vi "UI_PC event.vi"() -> ()   [LabVIEW 2016]
panel:
  out "RT TCP Loop time 3":u32
  out "RT TCP Loop time 2":u32
  out "RT TCP Loop time":u32
  in  "latch":bool
  in  "type 2":T1
  in  "switch":bool
  in  "정지":bool
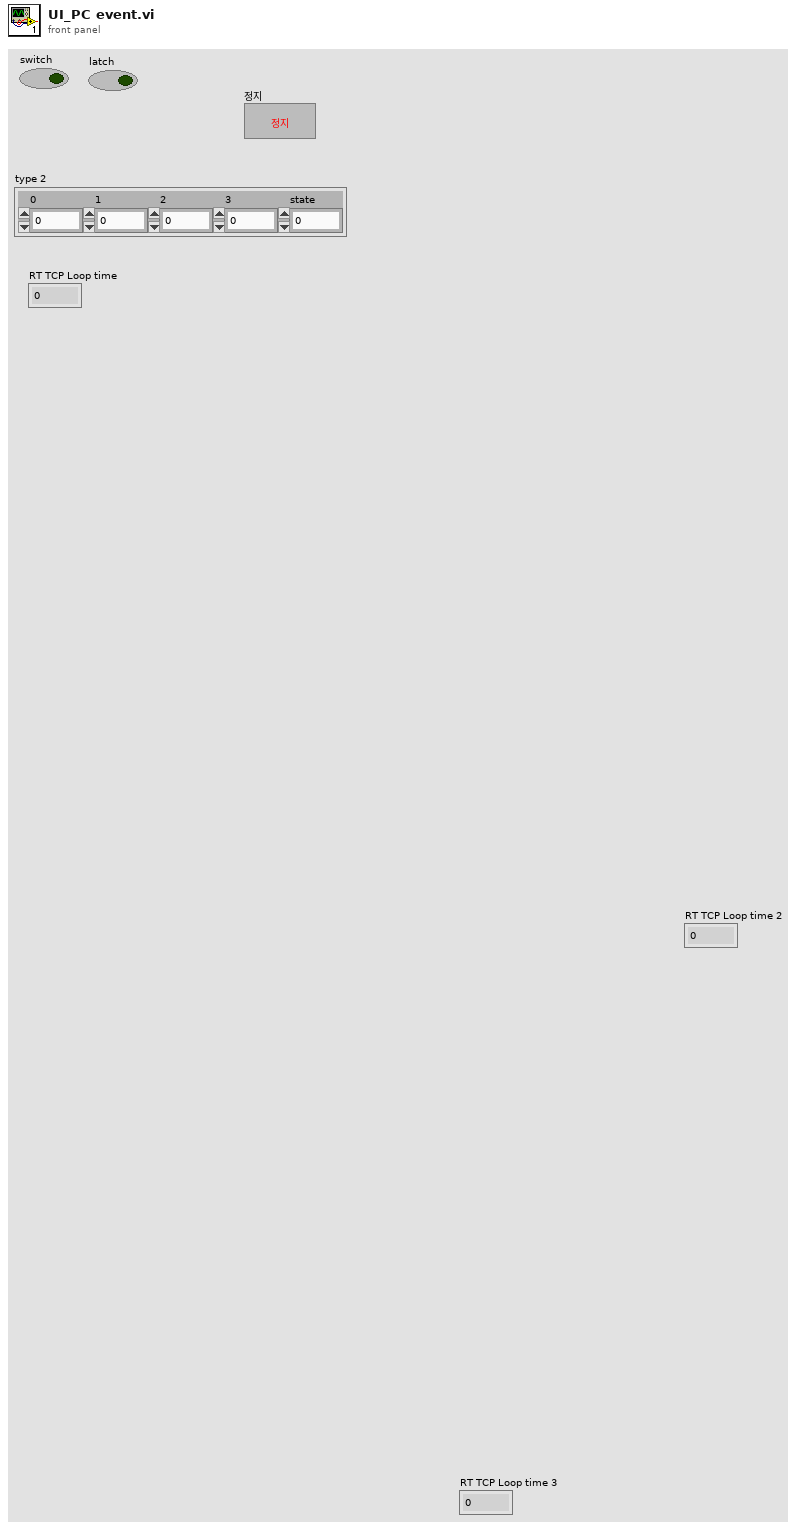
[diagram p1: front panel]
types:
  T1 = cluster{"0":sgl, "1":sgl, "2":sgl, "3":sgl, "state":i32}
  T2 = enum16{"big-endian, network order", "native, host order", "little-endian"}
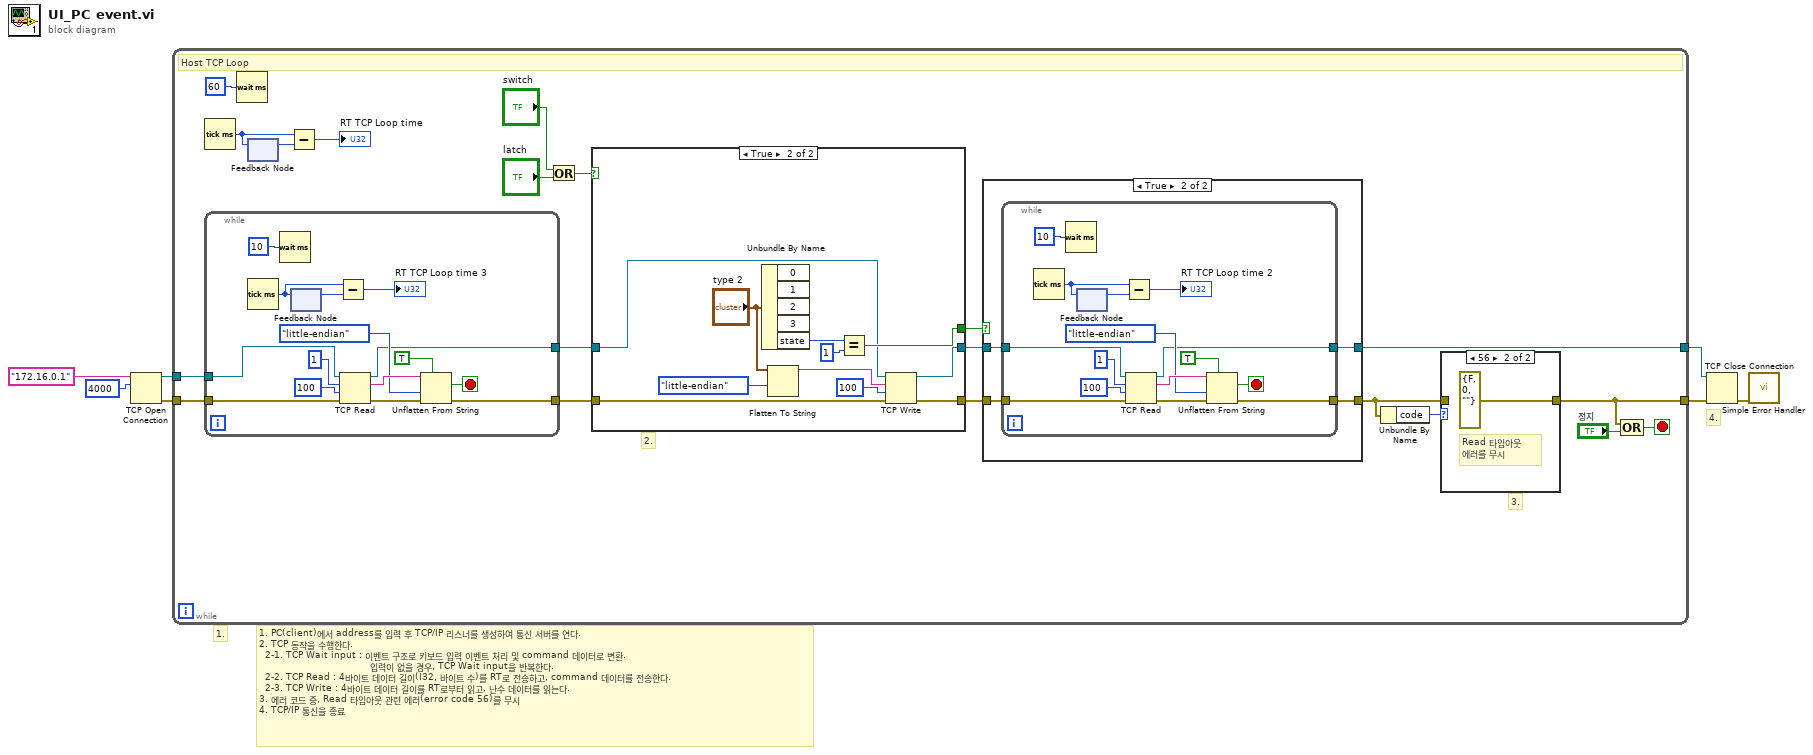
[diagram p0: block diagram]
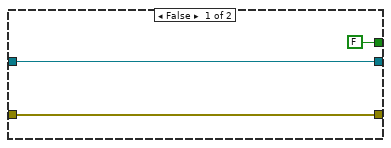
[diagram p3: hidden frame]
diagram:
  # "1. PC(client)에서 address를 입력 후 TCP/IP 리스너를 생성하여 통신 서버를 연다.\n2. TCP 동작을 수행한다.\n  2-1. TCP Wait input : 이벤트 구조로 키보드 입력 이벤트 처리 및 command 데이터로 변환.\n                                     입력이 없을 경우, TCP Wait input을 반복한다.\n  2-2. TCP Read : 4바이트 데이터 길이(I32, 바이트 수)를 RT로 전송하고, command 데이터를 전송한다.\n  2-3. TCP Write : 4바이트 데이터 길이를 RT로부터 읽고, 난수 데이터를 읽는다.\n3. 에러 코드 중, Read 타임아웃 관련 에러(error code 56)를 무시\n4. TCP/IP 통신을 종료"
  # "4."
  # "1."
  n1 = TCP Open Connection(address="172.16.0.1" ("주소"), remote port or service name=u16 4000 ("원격 포트 또는 서비스 이름")) -> (connection ID=w7:refnum<k5>, error out=w4:errorcluster)  [unwired: 3 in]
  n2 = while {
    tunnel: w7 -> [w11]
    tunnel: w4 -> [w10]
    tunnel: [w15] -> w3
    tunnel: [w24] -> w2
    stop <- w26 stop-if-true
    # "2."
    # "3."
    # "Host TCP Loop"
    n3 = Tick Count (ms)() -> (millisecond timer value=w13:u32)
    n4 = while {
      tunnel: w11 -> [w42]
      tunnel: [w34] -> w8
      tunnel: w10 -> [w41]
      tunnel: [w28] -> w9
      stop <- w29 stop-if-true
      n5 = Tick Count (ms)() -> (millisecond timer value=w32:u32)
      n6 = Wait (ms)(milliseconds to wait=u32 10 ("대기 시간 (ms)")) -> ()  [unwired: 1 out]
      n7 = feedback #1() -> (w33:u32)  [unwired: 1 in]
      n8 = feedback-in #1(w32) -> ()
      n9 = Subtract(x=w32, y=w33) -> (x-y=→"RT TCP Loop time 3":u32)
      n10 = TCP Read(connection ID=w42, bytes to read=1, error in (no error)=w41, 9:100 ("타임아웃 ms (25000)")) -> (connection ID out=w34:refnum<k5>, data out=w38:string, error out=w35:errorcluster)  [unwired: 1 in]
      n11 = Unflatten From String(type=TRUE, binary string=w38, byte order (0:big-endian, network order)=T2."little-endian", error in (no error)=w35) -> (value=w29:bool, error out=w28:errorcluster)  [unwired: 1 in, 1 out]
    }
    n12 = Wait (ms)(milliseconds to wait=u32 60 ("대기 시간 (ms)")) -> ()  [unwired: 1 out]
    n13 = feedback #2() -> (w14:u32)  [unwired: 1 in]
    n14 = feedback-in #2(w13) -> ()
    n15 = Subtract(x=w13, y=w14) -> (x-y=→"RT TCP Loop time":u32)
    n16 = Or(x="switch", y="latch") -> (x .or. y?=w21:bool)
    n17 = case shown="True" w21 {
      tunnel: w9 -> [w66 w77]
      tunnel: [w64 w74] -> w18
      tunnel: [w66 w73] -> w17
      tunnel: [FALSE w68] -> w19
      tunnel: w8 -> [w64 w67]
      frame False {
      }
      frame True {
        n18 = Unbundle By Name("type 2") -> ("state"=w70:i32)  [unwired: 4 out]
        n19 = Flatten To String(anything="type 2", byte order (0:big-endian, network order)=T2."little-endian") -> (data string=w76:string)  [unwired: 2 in, 2 out]
        n20 = Equal?(x=w70, y=1) -> (x = y?=w68:bool)
        n21 = TCP Write(connection ID=w67, data in=w76, error in (no error)=w77, 9:100 ("timeout ms (25000)")) -> (connection ID out=w74:refnum<k5>, error out=w73:errorcluster)  [unwired: 1 out]
      }
    }
    n22 = case shown="True" w19 {
      tunnel: w18 -> [w44 w48]
      tunnel: w17 -> [w43 w47]
      tunnel: [w43 w46] -> w16
      tunnel: [w44 w45] -> w15
      frame False {
      }
      frame True {
        n23 = while {
          tunnel: w48 -> [w63]
          tunnel: w47 -> [w62]
          tunnel: [w55] -> w46
          tunnel: [w54] -> w45
          stop <- w49 stop-if-true
          n24 = Tick Count (ms)() -> (millisecond timer value=w52:u32)
          n25 = Wait (ms)(milliseconds to wait=u32 10 ("대기 시간 (ms)")) -> ()  [unwired: 1 out]
          n26 = feedback #3() -> (w53:u32)  [unwired: 1 in]
          n27 = feedback-in #3(w52) -> ()
          n28 = Subtract(x=w52, y=w53) -> (x-y=→"RT TCP Loop time 2":u32)
          n29 = TCP Read(connection ID=w63, bytes to read=1, error in (no error)=w62, 9:100 ("타임아웃 ms (25000)")) -> (connection ID out=w54:refnum<k5>, data out=w59:string, error out=w56:errorcluster)  [unwired: 1 in]
          n30 = Unflatten From String(type=TRUE, binary string=w59, byte order (0:big-endian, network order)=T2."little-endian", error in (no error)=w56) -> (value=w49:bool, error out=w55:errorcluster)  [unwired: 1 in, 1 out]
        }
      }
    }
    n31 = Unbundle By Name(w16) -> ("code"=w25:i32)
    n32 = case shown="56" w25 {
      tunnel: [w78 errorcluster {"status"=FALSE, "code"=0, "source"=""} ("에러 출력")] -> w24
      tunnel: w16 -> [w78 _]
      frame 0, Default {
      }
      frame 56 {
        # "Read 타임아웃\n에러를 무시"
      }
    }
    n33 = Compound Arithmetic op=OR ("복합 연산")(w24, "정지") -> (w26:bool)
  }
  n34 = TCP Close Connection(connection ID=w3, error in (no error)=w2) -> (error out=w1:errorcluster)  [unwired: 1 in, 1 out]
  n35 = call <vilib>:"Simple Error Handler.vi"("error in (no error)"=w1) -> ()  [unwired: 4 in, 5 out]
